vi "Normalization.vi"(11 "x":dbl) -> (2 "Normalization":dbl)   [LabVIEW 2020]
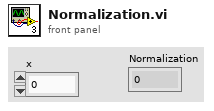
[diagram p1: front panel]
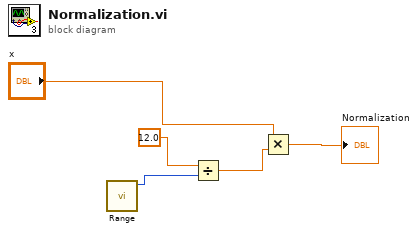
[diagram p0: block diagram]
diagram:
  n1 = call "Range.vi"() -> ("NumBins"=w4:i32)  [unwired: 10 in, 1 out]
  n2 = Divide(x=12.0, y=w4) -> (x/y=w3:dbl)
  n3 = Multiply(x="x", y=w3) -> (x*y=→"Normalization":dbl)
